vi "TI-SigmaGraph.vi"(6 "TI bounds":T4, 7 "sigma/U bounds":T4, 8 "UnderlayPlotSeries":string[](array[string]), 9 "Pre-plot Injection":string, 10 "gnuplotIn":string, 11 "Basics Visible":bool[](array[boolean])) -> (2 "gnuplotOut":string)   [LabVIEW 2015]
uses:
  minAndMax.ctl
  AutoManualNumber.ctl
  ticsAndGrids.ctl
  tics.ctl
  grids.ctl
  axisName.ctl
panel:
  in  "SigmaPlot":string="FILE index 3 using 1:(jittered($2)) axes x2y1 title 'sigma/U' w points lc rgb '#800000' pt 2 ps 0.8"
  in  "TIlplot":string="FILE index 2 using 1:(jittered($2)) axes x1y1 title 'Turbulence' w points lc rgb '#000080' pt 6 ps 1.5"
  in  "SigmaLabelAndTics":string="# X2 label (Hand-positioned, so it can inclue \"point\" command, and using previously defined colours \"b\" and \"g\"):\nset label '\\footnotesize \\color{t}{$\\sigma(U)/U_{ref}$}' offset 1,-0.2 point lc rgb \"#800000\" pt 2 ps 0.8 at graph 0.35, 1.08\nset x2tics format '\\footnotesize \\color{t}$%g$' offset 0,-0.5"
  in  "TIlabelAndTics":string="# X1 label (Hand-positioned, so it can inclue \"point\" command, and using previously defined colours \"b\" and \"g\"):\nset label '\\color{b}{$Turbulence~Intensity, \\sigma(U)/\\overline{U}$~(\\%)}' offset 1,-0.2 point lc rgb \"#000080\" pt 6 ps 1.5 at graph 0.15, -0.1\nset xtics format '\\color{b}$%g$'"
  in  "SigmaTicsAndGrids":T1={"tics"={"ticMin"=0.0, "ticStep"=0.02, "ticMax"=0.1, "minorDivsPerMajor"=2, "ticSpacing"=enum."Auto Tics", "ticPosition"=enum."Outside, no mirror"}, "Grids"={"Gridlines"=enum."No grids", "Zeroaxis"=enum."No zero axis"}, "Mapping"=enum."Lin"}
  in  "TurbulenceTicsAndGrids":T1={"tics"={"ticMin"=0.0, "ticStep"=5.0, "ticMax"=30.0, "minorDivsPerMajor"=2, "ticSpacing"=enum."Auto Tics", "ticPosition"=enum."Outside, no mirror"}, "Grids"={"Gridlines"=enum."Major grid", "Zeroaxis"=enum."No zero axis"}, "Mapping"=enum."Lin"}
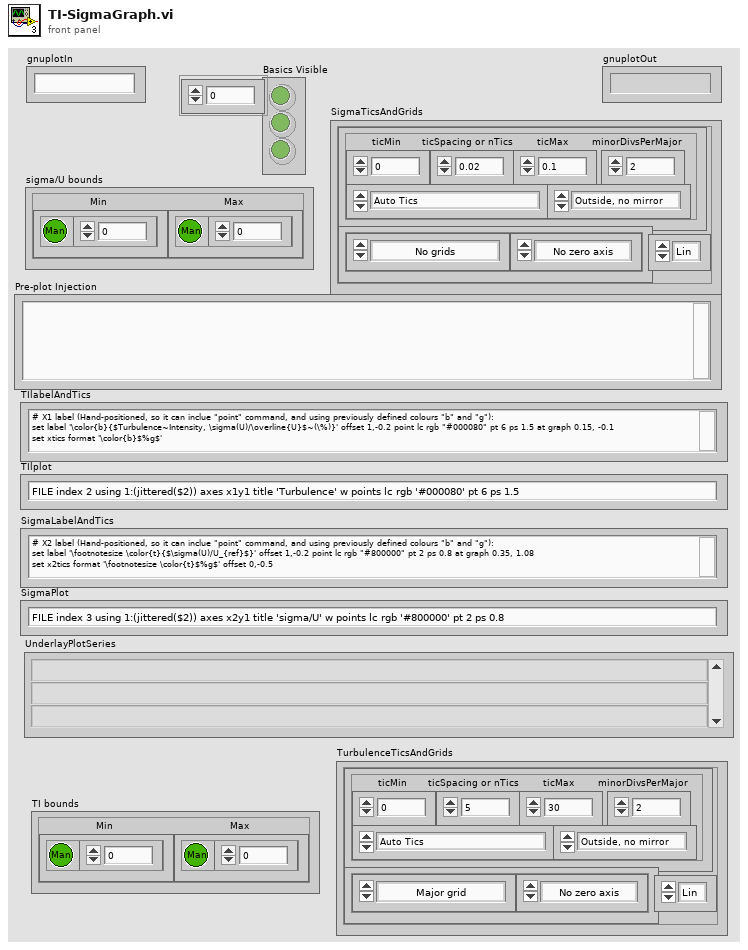
[diagram p1: front panel]
types:
  T1 = typedef "ticsAndGrids.ctl" = cluster{"tics":T2, "Grids":T3, "Mapping":enum8{"Lin", "Log"}}
  T2 = typedef "tics.ctl" = cluster{"ticMin":dbl, "ticStep":dbl, "ticMax":dbl, "minorDivsPerMajor":i32, "ticSpacing":enum16{"Auto Tics", "Fixed spacing", "Fixed Minimum and Spacing", "Start, Spacing and Maximum", "Approx n Tics (rounded)"}, "ticPosition":enum16{"Inside, no mirror", "Inside, mirrored", "Outside, no mirror", "Outside, mirrored", "Invisible"}}
  T3 = typedef "grids.ctl" = cluster{"Gridlines":enum16{"No grids", "Major grid", "Minor grid", "Major and Minor"}, "Zeroaxis":enum16{"No zero axis", "Show zero axis"}}
  T4 = typedef "minAndMax.ctl" = cluster{"Min":T5, "Max":T5}
  T5 = typedef "AutoManualNumber.ctl" = cluster{"Auto":bool, "Value":dbl}
  T6 = typedef "axisName.ctl" = string
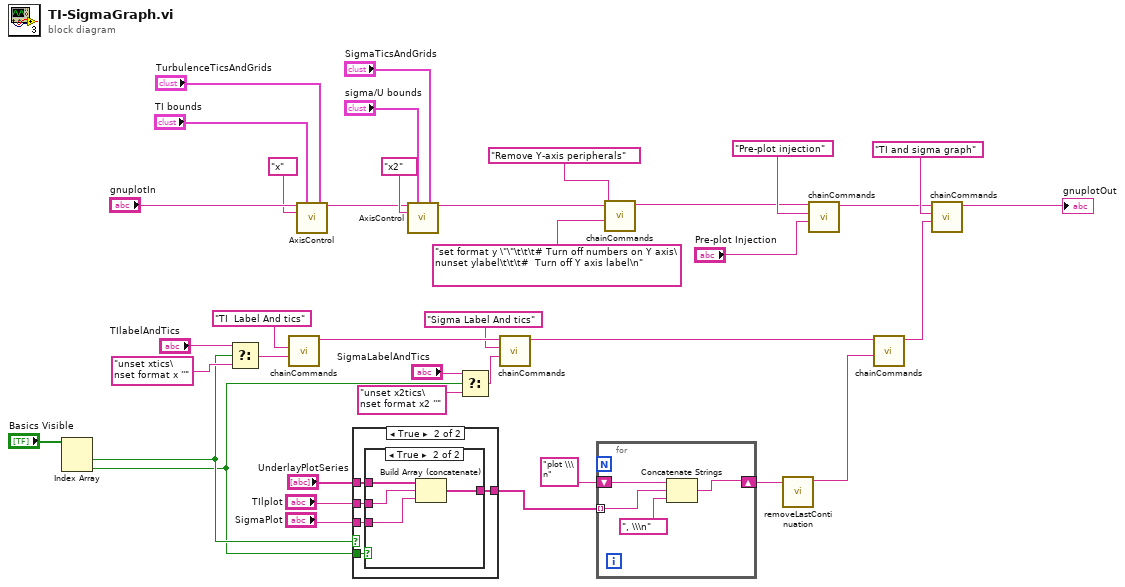
[diagram p0: block diagram]
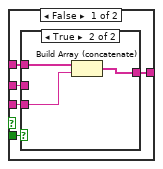
[diagram p2: hidden frame]
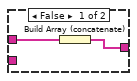
[diagram p3: hidden frame]
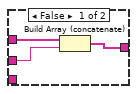
[diagram p4: hidden frame]
diagram:
  n1 = Index Array(array="Basics Visible") -> (element #1=w13:bool, element #2=w12:bool)  [unwired: 2 in]
  n2 = Select(t="TIlabelAndTics", s=w13, f="unset xtics\nset format x ''") -> (s? t:f=w17:string)
  n3 = call "chainCommands.vi"("Command"=w17, "Comments"="TI  Label And tics" ("Preamble")) -> ("StringOut"=w22:string)  [unwired: 9 in]
  n4 = call "AxisControl.vi"("String in"="gnuplotIn", "AxisBounds"="TI bounds", "ticsAndGrids"="TurbulenceTicsAndGrids", "Axis"=T6 "x") -> ("String out"=w33:string)  [unwired: 10 in, 1 out]
  n5 = case shown="True" w13 {
    tunnel: "UnderlayPlotSeries" -> [w43 w53]
    tunnel: [w42 w52] -> w25
    tunnel: "TIlplot" -> [w41 w51]
    tunnel: "SigmaPlot" -> [w40 w50]
    tunnel: w12 -> [w39 w49]
    frame False {
      n6 = case shown="True" w39 {
        tunnel: w43 -> [w45 w48]
        tunnel: [w44 w47] -> w42
        tunnel: w41 -> [_ _]
        tunnel: w40 -> [_ w46]
        frame False {
          n7 = Build Array (concatenate)(w45) -> (w44:string[])
        }
        frame True {
          n8 = Build Array (concatenate)(w48, w46) -> (w47:string[])
        }
      }
    }
    frame True {
      n9 = case shown="True" w49 {
        tunnel: w53 -> [w56 w60]
        tunnel: [w55 w59] -> w52
        tunnel: w51 -> [w54 w58]
        tunnel: w50 -> [_ w57]
        frame False {
          n10 = Build Array (concatenate)(w56, w54) -> (w55:string[])
        }
        frame True {
          n11 = Build Array (concatenate)(w60, w58, w57) -> (w59:string[])
        }
      }
    }
  }
  n12 = call "AxisControl.vi"("String in"=w33, "AxisBounds"="sigma/U bounds", "ticsAndGrids"="SigmaTicsAndGrids", "Axis"=T6 "x2") -> ("String out"=w4:string)  [unwired: 10 in, 1 out]
  n13 = Select(t="SigmaLabelAndTics", s=w12, f="unset x2tics\nset format x2 ''") -> (s? t:f=w14:string)
  n14 = call "chainCommands.vi"("Command"=w14, "Comments"="Sigma Label And tics" ("Preamble"), "StringIn"=w22) -> ("StringOut"=w21:string)  [unwired: 8 in]
  n15 = for {
    tunnel: w25 -> [w64] mode=indexing
    shift-right: [w61] -> w24
    shift-left: "plot \\\n" -> [w62]
    n16 = Concatenate Strings(w62, w64, ", \\\n" ("string")) -> (w61:string)
  }
  n17 = call "chainCommands.vi"("Command"="set format y \"\"\t\t\t# Turn off numbers on Y axis\nunset ylabel\t\t\t#  Turn off Y axis label\n" ("CoreCommand"), "Comments"="Remove Y-axis peripherals", "StringIn"=w4) -> ("StringOut"=w3:string)  [unwired: 8 in]
  n18 = call "removeLastContinuation.vi"("String in"=w24) -> ("String out"=w20:string)  [unwired: 10 in]
  n19 = call "chainCommands.vi"("Command"="Pre-plot Injection", "Comments"="Pre-plot injection", "StringIn"=w3) -> ("StringOut"=w26:string)  [unwired: 8 in]
  n20 = call "chainCommands.vi"("Command"=w20, "StringIn"=w21) -> ("StringOut"=w11:string)  [unwired: 9 in]
  n21 = call "chainCommands.vi"("Command"=w11, "Comments"="TI and sigma graph", "StringIn"=w26) -> ("StringOut"=→"gnuplotOut":string)  [unwired: 8 in]
